vi "Header Licor-Data.vi"(7 "Licor-Sources":T1[](array[typedef])) -> (8 "Header":string[](array[string]))   [LabVIEW 2010, in "Licor-Steuerung.lvlib"]
uses:
  Licor-Steuerung.lvlib
  LicorLI7000/conventions/Licor-Source.ctl
  util/util.lvlib
  LicorLI7000/LicorLI7000.lvlib
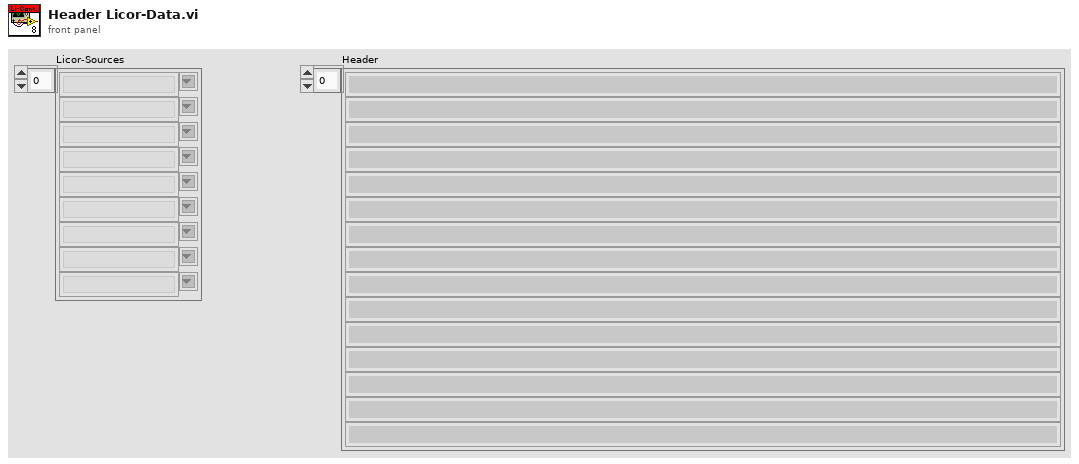
[diagram p1: front panel]
types:
  T1 = typedef "LicorLI7000.lvlib/Licor-Source.ctl" = string
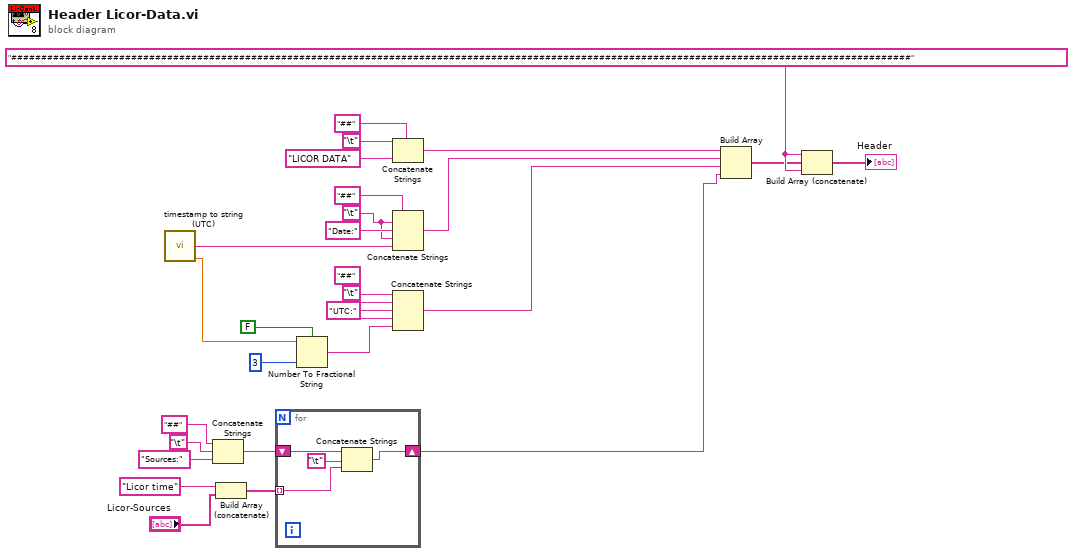
[diagram p0: block diagram]
diagram:
  w10 = "\t"
  w14 = "\t"
  w28 = "######################################################################################################################################################"
  n1 = call "timestamp to string (UTC).vi"() -> ("date/time string (UTC)"=w5:string, "UTC [s]"=w4:dbl)  [unwired: 14 in]
  n2 = Concatenate Strings("##", "\t", "Sources:") -> (w22:string)
  n3 = Build Array (concatenate)("Licor time" ("group name"), "Licor-Sources") -> (w2:T1[])
  n4 = for {
    tunnel: w2 -> [w30] mode=indexing
    shift-right: [w29] -> w13
    shift-left: w22 -> [w32]
    n5 = Concatenate Strings(w32, "\t", w30) -> (w29:string)
  }
  n6 = Number To Fractional String(use system decimal point (T)=FALSE ("Systemdezimalzeichen verwenden (T)"), number=w4, precision (6)=i16 3 ("Genauigkeit (6)")) -> (F-format string=w8:string)  [unwired: 1 in]
  n7 = Concatenate Strings("##", "\t", "LICOR DATA") -> (w18:string)
  n8 = Concatenate Strings("##", w14, "Date:" ("String"), w14, w5) -> (w16:string)
  n9 = Concatenate Strings("##", w10, "UTC:" ("String"), w10, w8) -> (w7:string)
  n10 = Build Array(w18, w16, w7, w13) -> (w27:string[])
  n11 = Build Array (concatenate)(w28, w27, w28) -> (→"Header":string[])
